vi "BrowseCallData.vi"() -> ()   [LabVIEW 2022 SP3]
uses:
  <vilib>/Analysis/4window.llb/Hamming Window (DBL).vi
  <vilib>/Analysis/baseanly.llb/Quick Scale 1D.vi
  <vilib>/Analysis/4window.llb/AllCosWindow (DBL).vi
  <vilib>/Utility/file.llb/Read From Spreadsheet File (DBL).vi
  <vilib>/Analysis/2dsp.llb/Zero Padder (DBL).vi
  <vilib>/Analysis/NI_AALPro.lvlib
  <vilib>/Analysis/NI_AALBase.lvlib
panel:
  out "time trace":dbl[](graph)
  out "path":path
  in  "Boolean":bool
  out "all rows 2":dbl[][](array[numeric]) format="%0.3f"
  out "Power spectrum":T1(graph)
  out "F step time":dbl
  in  "v step":u16
  out "Voltage step time":dbl
  out "all rows":dbl[][](array[numeric]) format="%0.3f"
  out "Pressure curve 2":cluster{"all rows":dbl[], "all rows":dbl[]}(graph)
  out "Pressure curve":cluster{"all rows":dbl[], "all rows":dbl[]}(graph)
  out "f (MHZ)":dbl
  in  "F step":u16
  in  "stop":bool
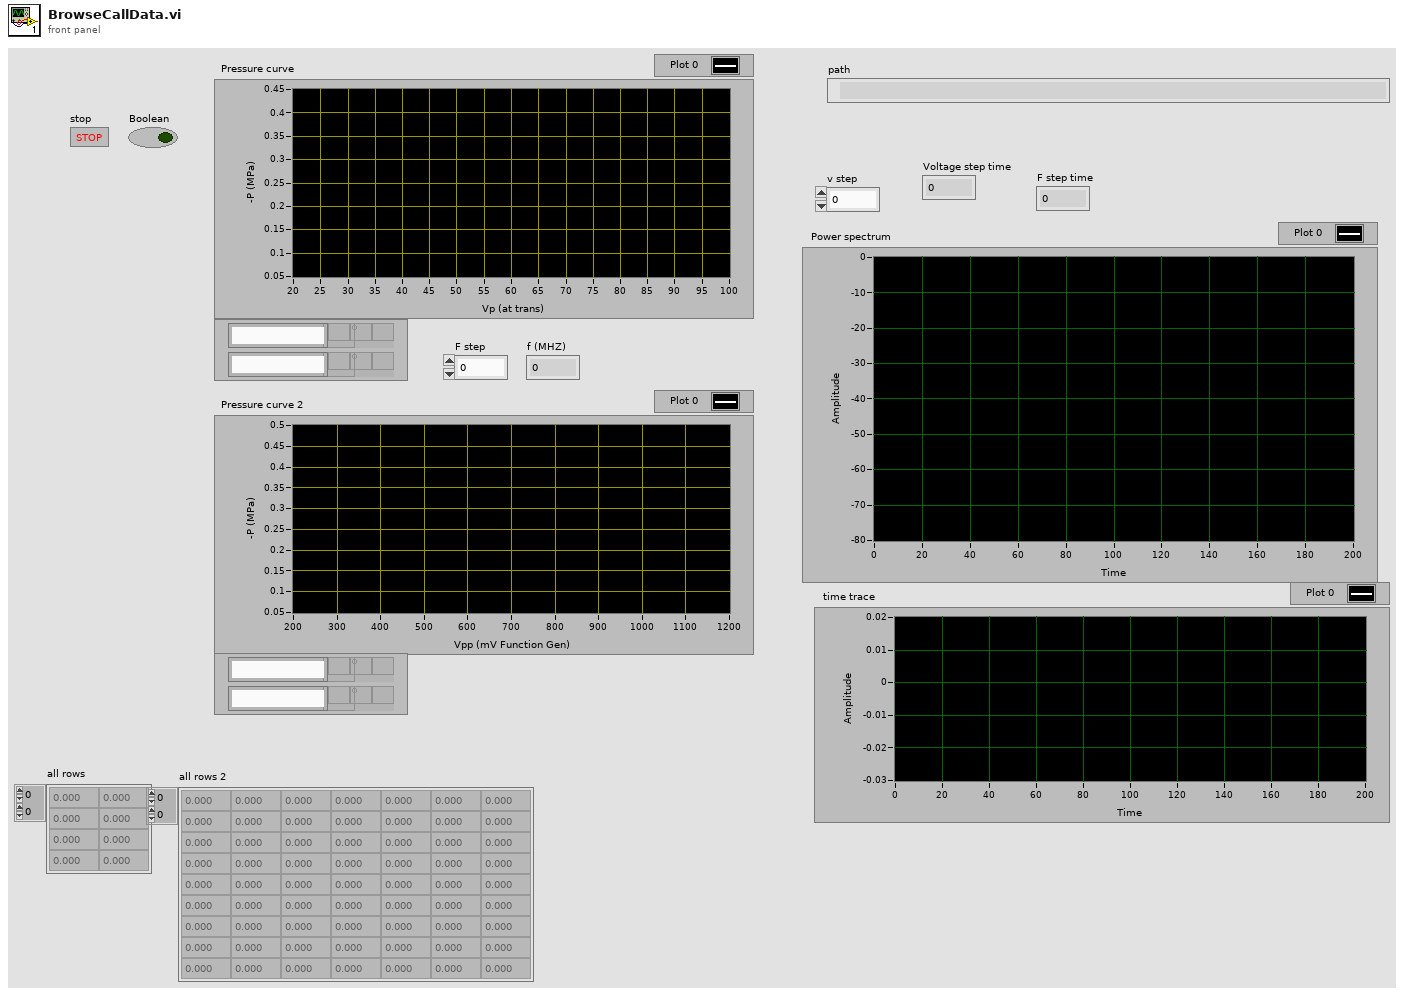
[diagram p1: front panel]
types:
  T1 = cluster{"df":dbl, "df":dbl, "Power Spectrum (V^2 rms)":dbl[]}
  T2 = cluster{"df":dbl, "df":dbl, "Y[i]=X[i]/Max|X|":dbl[]}
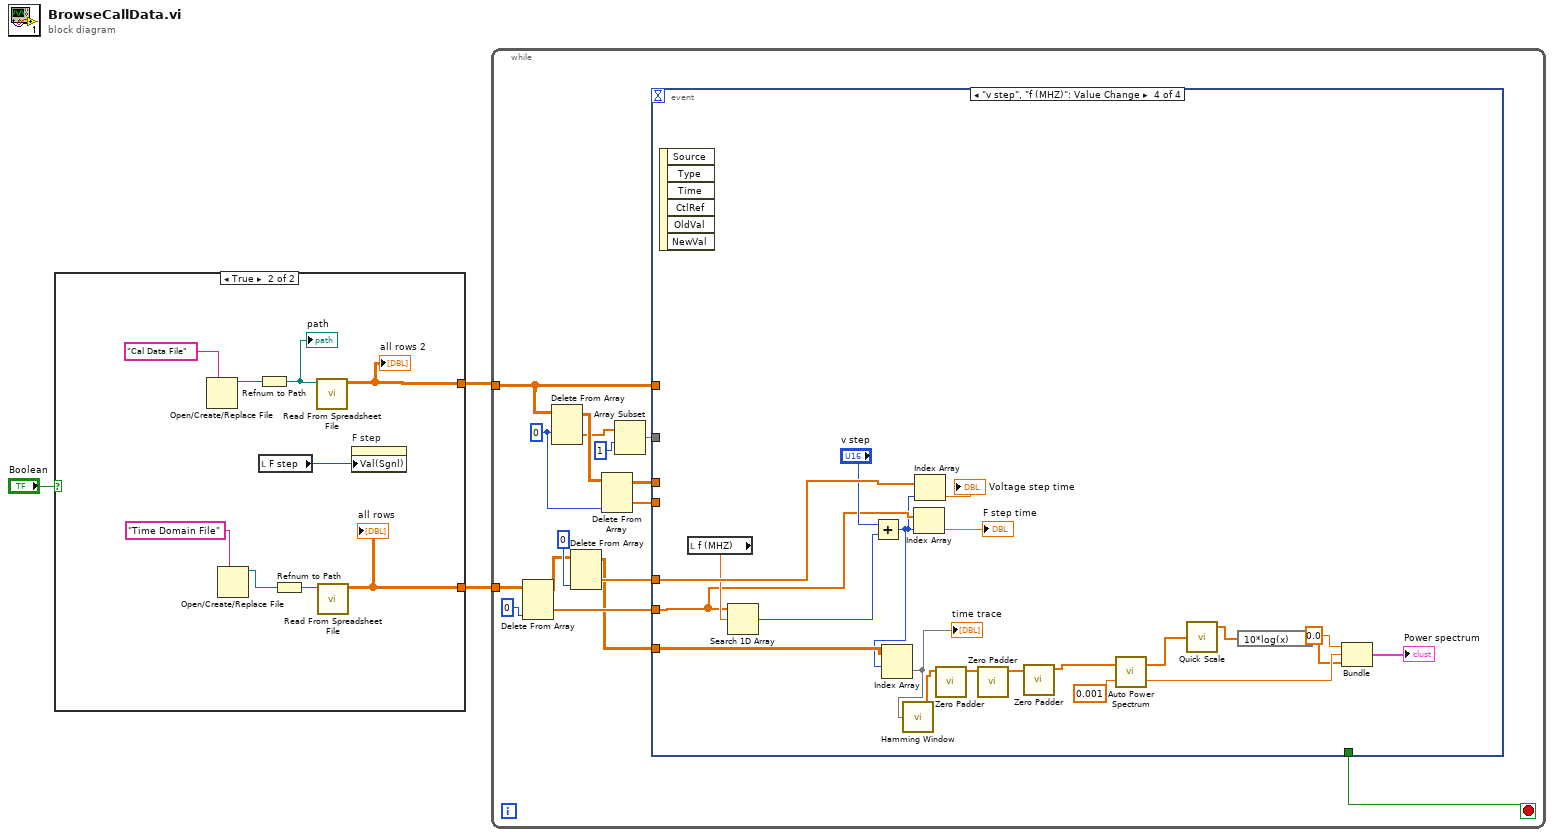
[diagram p0: block diagram]
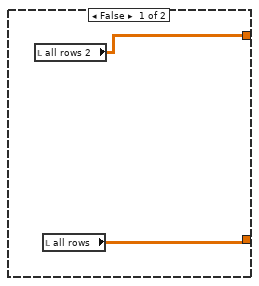
[diagram p2: hidden frame]
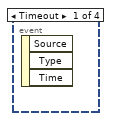
[diagram p3: hidden frame]
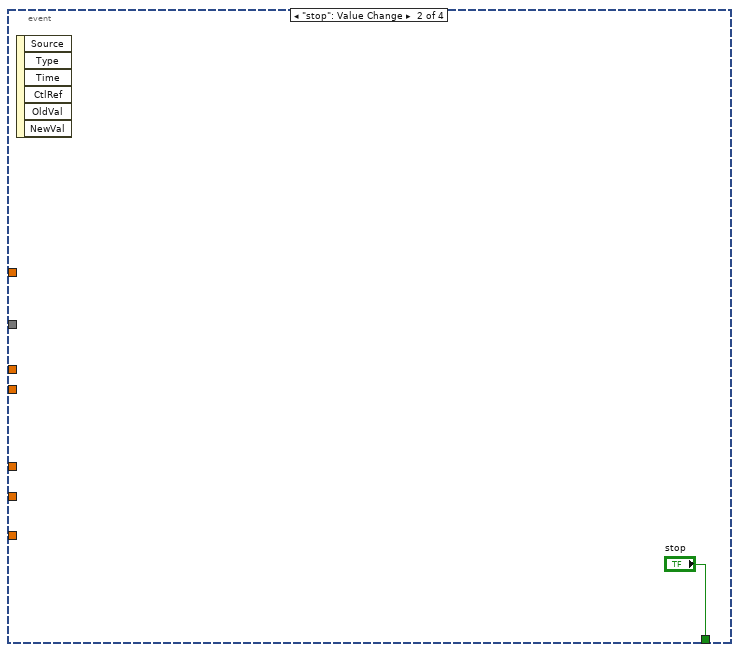
[diagram p4: hidden frame]
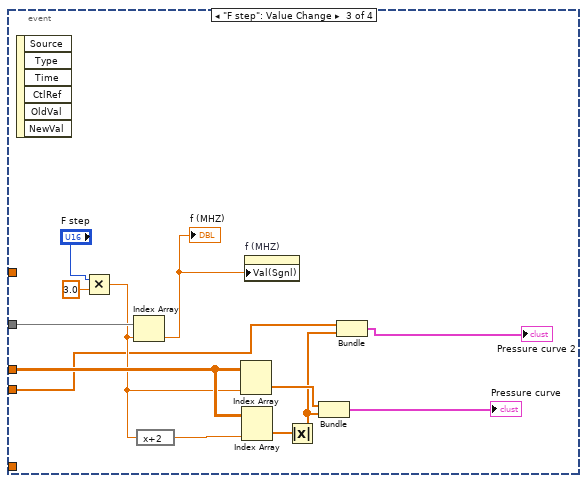
[diagram p5: hidden frame]
diagram:
  n1 = case shown="True" "Boolean" {
    tunnel: [w4 w7] -> w3
    tunnel: [w5 w8] -> w2
    frame False {
      n2 = local read "all rows 2"() -> (w4:dbl[][])
      n3 = local read "all rows"() -> (w5:dbl[][])
    }
    frame True {
      n4 = Open/Create/Replace File(prompt="Cal Data File") -> (refnum out=w14:refnum<file>)  [unwired: 5 in, 2 out]
      n5 = Open/Create/Replace File(prompt="Time Domain File") -> (refnum out=w11:refnum<file>)  [unwired: 5 in, 2 out]
      n6 = Refnum to Path(1:w14) -> (0:w13:path)
      "path" <- w13
      n7 = local read "F step"() -> (w6:u16)
      n8 = Refnum to Path(1:w11) -> (0:w10:path)
      n9 = call-poly <vilib>:"Read From Spreadsheet File.vi"("file path (dialog if empty)"=w13) -> ("all rows"=w7:dbl[][])  [unwired: 6 in, 4 out]
      "all rows 2" <- w7
      n10 = call-poly <vilib>:"Read From Spreadsheet File.vi"("file path (dialog if empty)"=w10) -> ("all rows"=w8:dbl[][])  [unwired: 6 in, 4 out]
      "all rows" <- w8
      n11 = property on="F step" class="DigNum (strict)"("Val(Sgnl)"=w6) -> ()  [unwired: 2 in, 2 out]
    }
  }
  n12 = while {
    tunnel: w3 -> [w29]
    tunnel: w2 -> [w21]
    stop <- w30 stop-if-true
    w27 = 0 ("index (row)")
    n13 = Delete From Array(array=w21, index (col)=0 ("index (row)")) -> (deleted portion=w16:dbl[], array with subset deleted=w18:dbl[][])  [unwired: 2 in]
    n14 = Delete From Array(array=w29, index (row)=w27) -> (deleted portion=w24:dbl[], array with subset deleted=w28:dbl[][])  [unwired: 2 in]
    n15 = Delete From Array(array=w18, index (col)=0 ("index (row)")) -> (deleted portion=w17:dbl[], array with subset deleted=w15:dbl[][])  [unwired: 2 in]
    n16 = Delete From Array(array=w28, index (col)=w27) -> (deleted portion=w25:dbl[], array with subset deleted=w26:dbl[][])  [unwired: 2 in]
    n17 = Array Subset(array=w24, index=1) -> (w22:dbl[])  [unwired: 1 in]
    n18 = event shown="[3] \"v step\", \"f (MHZ)\": Value Change" {
      selector: _ -> [_ _ _ _]
      dyn-events: _ -> [_ _ _ _]
      timeout: _ -> [_ _ _ _]
      tunnel: [_ "stop" _ _] -> w30
      tunnel: w29 -> [_ _ _ _]
      tunnel: w26 -> [_ _ w36 _]
      tunnel: w25 -> [_ _ w34 _]
      tunnel: w22 -> [_ _ w44 _]
      tunnel: w15 -> [_ _ _ w63]
      tunnel: w17 -> [_ _ _ w64]
      tunnel: w16 -> [_ _ _ w49]
      event Timeout {
        n19 = event-data() -> ()  [unwired: 1 in, 3 out]
      }
      event "stop": Value Change {
        n20 = event-data() -> ()  [unwired: 1 in, 6 out]
      }
      event "F step": Value Change {
        n21 = event-data() -> ()  [unwired: 1 in, 6 out]
        n22 = Multiply(x="F step", y=3.0) -> (x*y=w35:dbl)
        n23 = Index Array(array=w44, index=w35) -> (element=w32:dbl)
        "f (MHZ)" <- w32
        n24 = expression code="x+2"(w35) -> (w39:dbl)
        n25 = Index Array(array=w36, index (col)=w35) -> (element=w41:dbl[])  [unwired: 1 in]
        n26 = Index Array(array=w36, index (col)=w39) -> (element=w38:dbl[])  [unwired: 1 in]
        n27 = property on="f (MHZ)" class="DigNum (strict)"("Val(Sgnl)"=w32) -> ()  [unwired: 2 in, 2 out]
        n28 = Absolute Value(x=w38) -> (abs(x)=w37:dbl[])
        n29 = Bundle("all rows"=w41, w37) -> (→"Pressure curve":cluster{"all rows":dbl[], dbl[]})  [unwired: 1 in]
        n30 = Bundle("all rows"=w34, w37) -> (→"Pressure curve 2":cluster{"all rows":dbl[], dbl[]})  [unwired: 1 in]
      }
      event "v step", "f (MHZ)": Value Change {
        n31 = event-data() -> ()  [unwired: 1 in, 6 out]
        n32 = local read "f (MHZ)"() -> (w52:dbl)
        n33 = Search 1D Array(1D array=w49, element=w52) -> (index of element=w50:i32)  [unwired: 1 in]
        n34 = Add(x="v step", y=w50) -> (x+y=w47:i32)
        n35 = Index Array(array=w63, index (row)=w47) -> (element=w46:dbl[])  [unwired: 1 in]
        "time trace" <- w46
        n36 = call-poly <vilib>:"Hamming Window.vi"("X"=w46) -> ("Windowed X"=w45:dbl[])  [unwired: 1 out]
        n37 = Index Array(array=w49, index=w47) -> (element=→"F step time":dbl)
        n38 = Index Array(array=w64, index=w47) -> (element=→"Voltage step time":dbl)
        n39 = call-poly <vilib>:"Zero Padder.vi"("Input Array"=w45) -> ("Zero Padded Array"=w55:dbl[])  [unwired: 10 in]
        n40 = call-poly <vilib>:"Zero Padder.vi"("Input Array"=w55) -> ("Zero Padded Array"=w54:dbl[])  [unwired: 10 in]
        n41 = call-poly <vilib>:"Zero Padder.vi"("Input Array"=w54) -> ("Zero Padded Array"=w53:dbl[])  [unwired: 10 in]
        n42 = call <vilib>:"Auto Power Spectrum.vi"("dt"=0.001, "Signal (V)"=w53) -> ("df"=w61:dbl, "Power Spectrum (V^2 rms)"=w58:dbl[])
        n43 = call-poly <vilib>:"Quick Scale.vi"("X"=w58) -> ("Y[i]=X[i]/Max|X|"=w57:dbl[])  [unwired: 2 out]
        n44 = expression code="10*log(x)"(w57) -> (w56:dbl[])
        n45 = Bundle("df"=0.0, "df"=w61, "Y[i]=X[i]/Max|X|"=w56) -> (→"Power spectrum":T2)  [unwired: 1 in]
      }
    }
  }
